vi "4p1_HW_Task1_UCweesesr.vi"() -> ()   [LabVIEW 2016]
panel:
  out "Difference:":dbl
  in  "Water Refractive Index":dbl
  in  "Distance from Person to Tank":dbl
  in  "Perpendicular Distance from Tank to Fish":dbl
  in  "Thickness of Tank Walls":dbl
  in  "Tank Viewing Material Refraction Index":dbl
  in  "Air Refraction Index":dbl
  in  "Height":dbl
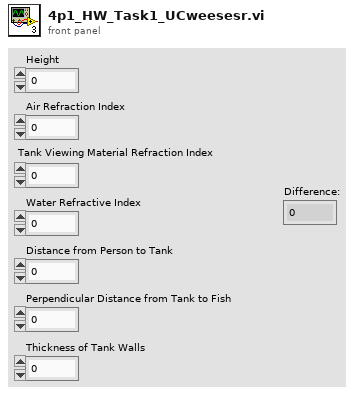
[diagram p1: front panel]
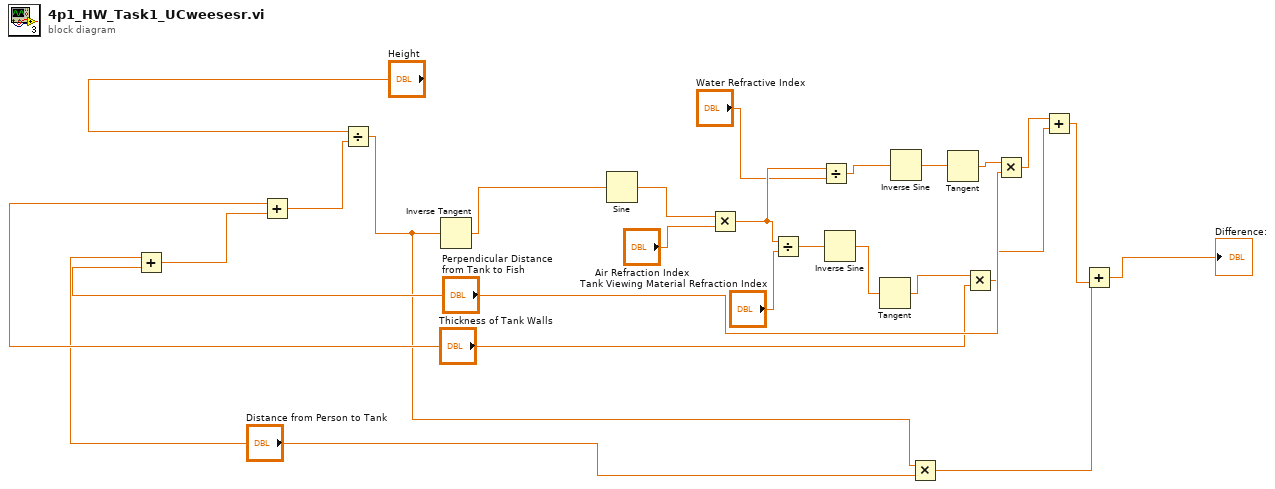
[diagram p0: block diagram]
diagram:
  n1 = Add(x="Distance from Person to Tank", y="Perpendicular Distance from Tank to Fish") -> (x+y=w24:dbl)
  n2 = Add(x="Thickness of Tank Walls", y=w24) -> (x+y=w22:dbl)
  n3 = Divide(x="Height", y=w22) -> (x/y=w2:dbl)
  n4 = Inverse Tangent(1:w2) -> (0:w1:dbl)
  n5 = Sine(x=w1) -> (sin(x)=w21:dbl)
  n6 = Multiply(x=w21, y="Air Refraction Index") -> (x*y=w17:dbl)
  n7 = Divide(x=w17, y="Tank Viewing Material Refraction Index") -> (x/y=w19:dbl)
  n8 = Divide(x=w17, y="Water Refractive Index") -> (x/y=w16:dbl)
  n9 = Inverse Sine(1:w19) -> (0:w15:dbl)
  n10 = Tangent(1:w15) -> (0:w12:dbl)
  n11 = Inverse Sine(1:w16) -> (0:w14:dbl)
  n12 = Multiply(x=w2, y="Distance from Person to Tank") -> (x*y=w4:dbl)
  n13 = Tangent(1:w14) -> (0:w13:dbl)
  n14 = Multiply(x=w12, y="Thickness of Tank Walls") -> (x*y=w7:dbl)
  n15 = Multiply(x=w13, y="Perpendicular Distance from Tank to Fish") -> (x*y=w6:dbl)
  n16 = Add(x=w6, y=w7) -> (x+y=w5:dbl)
  n17 = Add(x=w4, y=w5) -> (x+y=→"Difference:":dbl)
